vi "autofilter.vi"() -> ()   [LabVIEW 8.6]
uses:
  Controls/lxw_filter_criteria.ctl
  Controls/lxw_filter_operator.ctl
panel:
  out "error out":errorcluster
  out "function return 2":string
  # "autofilter.xlsx"
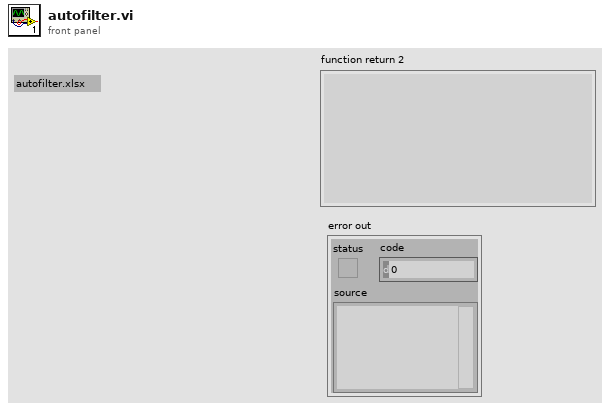
[diagram p1: front panel]
types:
  T1 = typedef "lxw_filter_operator.ctl" = u8
  T2 = typedef "lxw_filter_criteria.ctl" = u32
  T3 = cluster{"criteria":T2, "value_string":string, "value":dbl}
  T4 = cluster{"region":string[], "item":string[], "volume":i32[], "month":string[]}
  T5 = enum32{"invalid app kind", "Development System", "Run Time System", "Student Edition", "Embedded LabVIEW", "Evaluation", "Custom"}
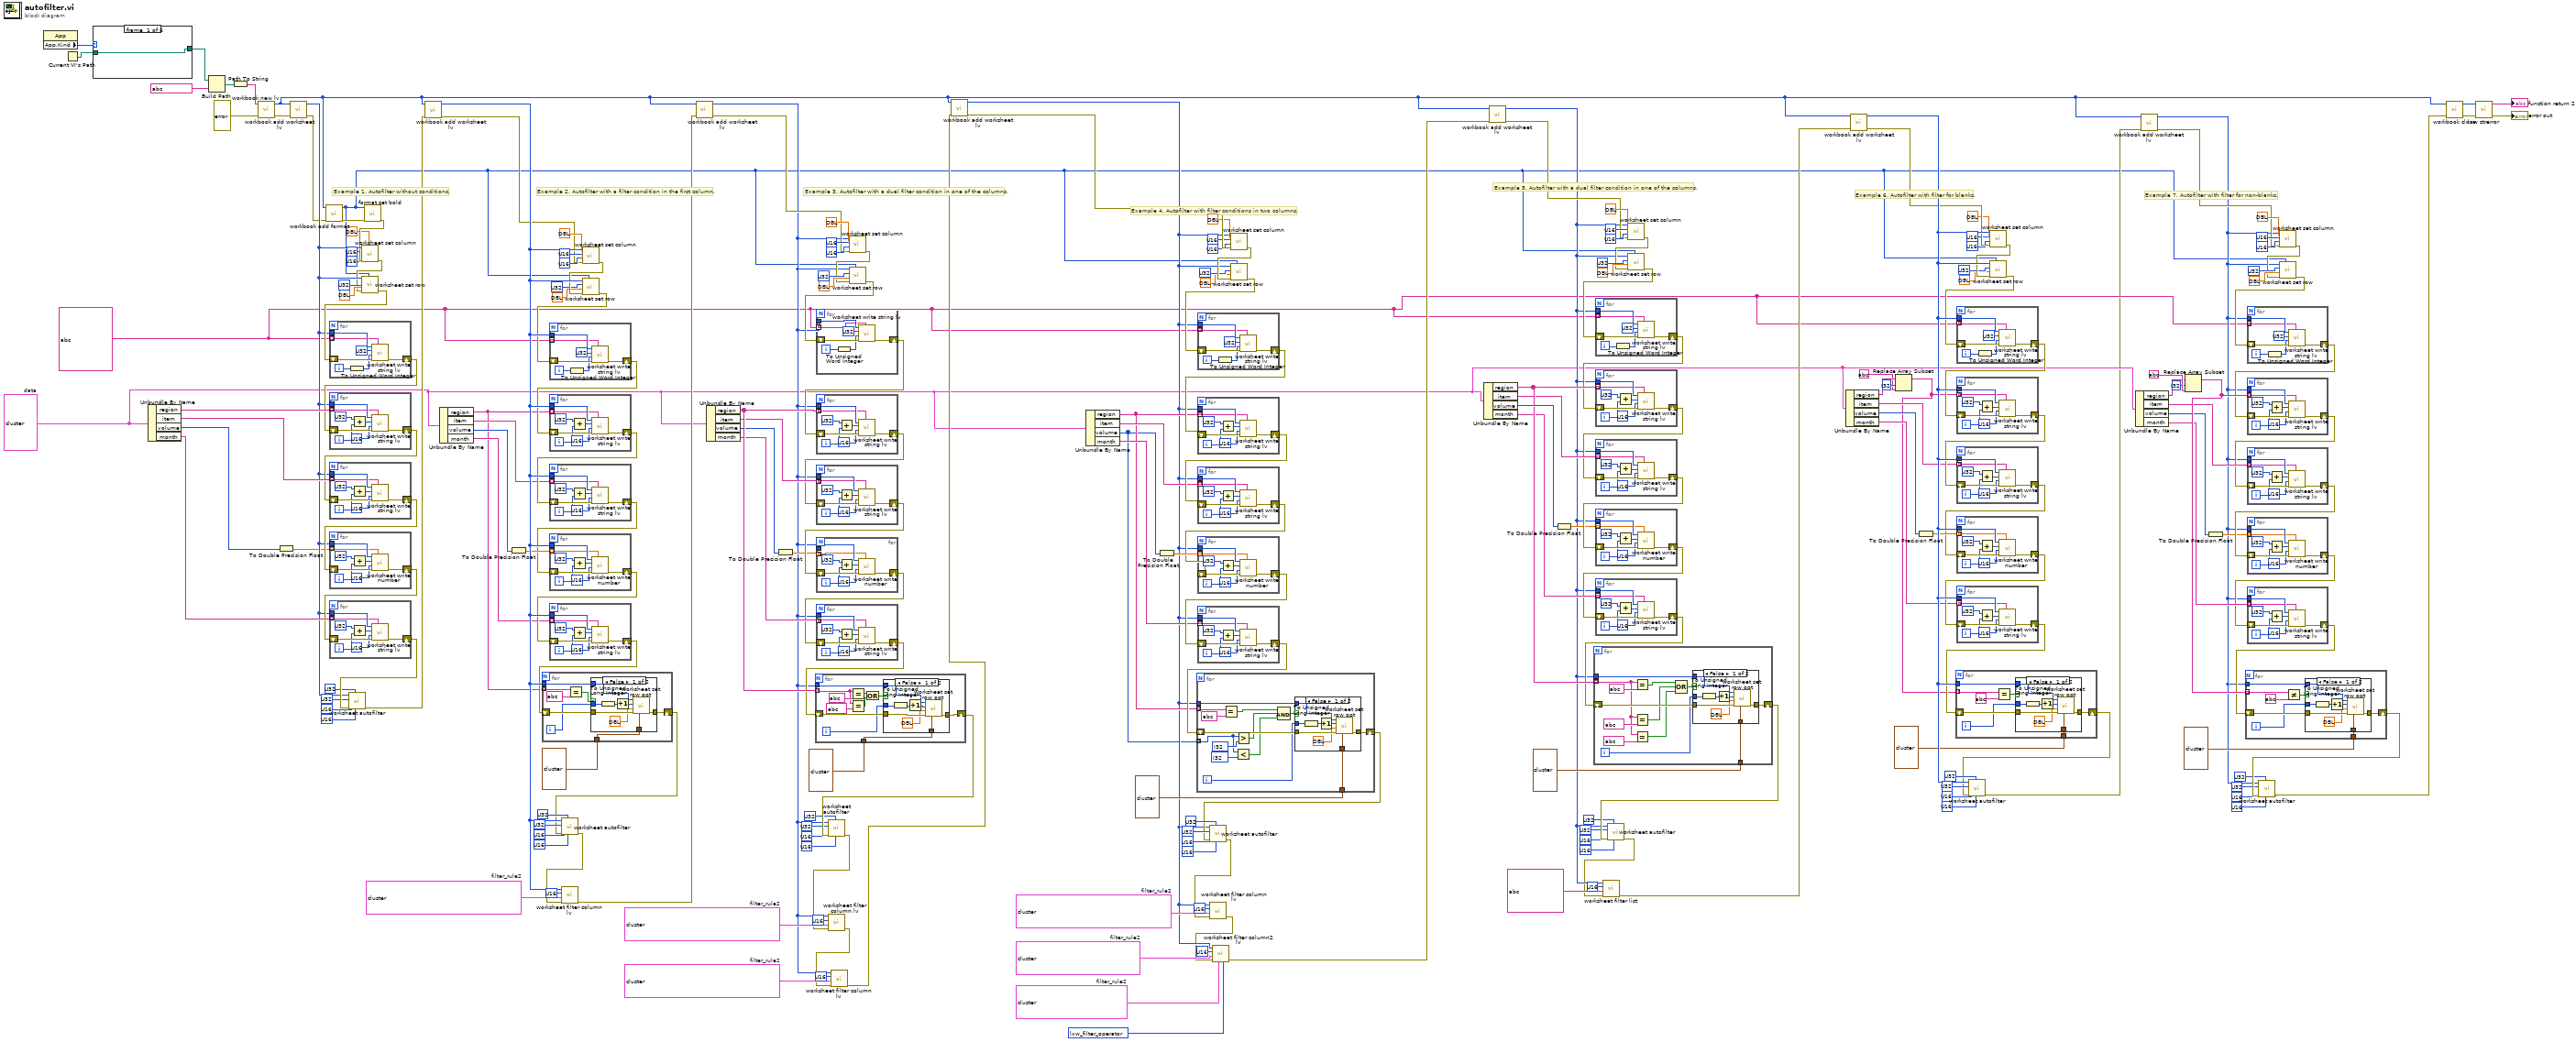
[diagram p0: block diagram]
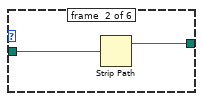
[diagram p8: hidden frame]
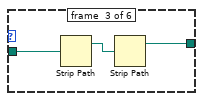
[diagram p9: hidden frame]
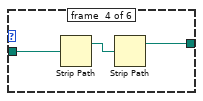
[diagram p10: hidden frame]
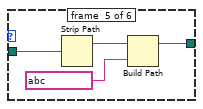
[diagram p11: hidden frame]
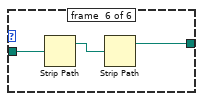
[diagram p12: hidden frame]
diagram:
  w95 = T1 ? items=["LXW_FILTER_AND", "LXW_FILTER_OR"] ("and_or")
  w97 = T3 ?  # filter_rule2
  w98 = T3 ?  # filter_rule2
  w103 = T3 ?  # filter_rule2
  w130 = T3 ?  # filter_rule2
  w155 = T3 ?  # filter_rule2
  w160 = T3 ?  # filter_rule2
  w5 = T4 ?  # data
  w6 = string[] ?
  # "Example 7. Autofilter with filter for non-blanks."
  # "Example 6. Autofilter with filter for blanks."
  # "Example 5. Autofilter with a dual filter condition in one of the columns."
  # "Example 4. Autofilter with filter conditions in two columns."
  # "Example 3. Autofilter with a dual filter condition in one of the columns."
  # "Example 2. Autofilter with a filter condition in the first column."
  # "Example 1. Autofilter without conditions."
  n1 = property class="App"() -> ("App.Kind"=w224:T5)  [unwired: 2 in, 2 out]
  n2 = Current VI's Path() -> (path=w223:path)
  n3 = case shown="\"Evaluation\"" w224 {
    tunnel: w223 -> [w225 w227 w230 w233 w237 w240]
    tunnel: [w225 w226 w228 w231 w235 w238] -> w222
    frame #0 {
    }
    frame #1 {
      n4 = Strip Path(path=w227) -> (stripped path=w226:path)  [unwired: 1 out]
    }
    frame #2 {
      n5 = Strip Path(path=w230) -> (stripped path=w229:path)  [unwired: 1 out]
      n6 = Strip Path(path=w229) -> (stripped path=w228:path)  [unwired: 1 out]
    }
    frame #3 {
      n7 = Strip Path(path=w233) -> (stripped path=w232:path)  [unwired: 1 out]
      n8 = Strip Path(path=w232) -> (stripped path=w231:path)  [unwired: 1 out]
    }
    frame #4 {
      n9 = Strip Path(path=w237) -> (stripped path=w236:path)  [unwired: 1 out]
      n10 = Build Path(base path=w236, name or relative path=string ?) -> (appended path=w235:path)
    }
    frame #5 {
      n11 = Strip Path(path=w240) -> (stripped path=w239:path)  [unwired: 1 out]
      n12 = Strip Path(path=w239) -> (stripped path=w238:path)  [unwired: 1 out]
    }
  }
  n13 = Unbundle By Name(w5) -> ("region"=w212:string[], "item"=w211:string[], "volume"=w202:i32[], "month"=w210:string[])
  n14 = Build Path(base path=w222, name or relative path=string ? ("filename")) -> (appended path=w214:path)
  n15 = Path To String(path=w214) -> (string=w213:string)
  n16 = call "workbook new lv.vi"("error in (no error)"=errorcluster ?, "filename"=w213) -> ("error out"=w220:errorcluster, "function return"=w4:u32)  [unwired: 8 in]
  n17 = To Double Precision Float(number=w202) -> (double precision float=w201:dbl[])
  n18 = call "workbook add worksheet lv.vi"("error in (no error)"=w220, "workbook"=w4) -> ("error out"=w199:errorcluster, "function return"=w203:u32)  [unwired: 8 in]
  n19 = call "workbook add format.vi"("error in (no error)"=w199, "workbook"=w4) -> ("error out"=w191:errorcluster, "function return"=w2:u32)  [unwired: 8 in]
  n20 = call "format set bold.vi"("error in (no error)"=w191, "format"=w2) -> ("error out"=w190:errorcluster)  [unwired: 9 in]
  n21 = call "worksheet set column.vi"("width"=dbl ?, "error in (no error)"=w190, "last_col"=u16 ?, "first_col"=u16 ?, "worksheet"=w203) -> ("error out"=w184:errorcluster)  [unwired: 5 in, 1 out]
  n22 = call "worksheet set row.vi"("format"=w2, "error in (no error)"=w184, "height"=dbl ?, "row"=u32 ?, "worksheet"=w203) -> ("error out"=w209:errorcluster)  [unwired: 5 in, 1 out]
  n23 = for {
    shift-right: [w247] -> w208
    shift-left: w209 -> [w246]
    tunnel: w203 -> [w245]
    tunnel: w6 -> [w244] mode=indexing
    i -> [w242]
    n24 = To Unsigned Word Integer(number=w242) -> (unsigned 16bit integer=w241:u16)
    n25 = call "worksheet write string lv.vi"("string"=w244, "error in (no error)"=w246, "col"=w241, "row"=u32 ?, "worksheet"=w245) -> ("error out"=w247:errorcluster)  [unwired: 5 in, 1 out]
  }
  n26 = for {
    shift-right: [w255] -> w207
    shift-left: w208 -> [w254]
    tunnel: w203 -> [w251]
    tunnel: w212 -> [w248] mode=indexing
    i -> [w250]
    n27 = Add(x=u32 ? ("row"), y=w250) -> (x+y=w253:u32)
    n28 = call "worksheet write string lv.vi"("string"=w248, "error in (no error)"=w254, "col"=u16 ?, "row"=w253, "worksheet"=w251) -> ("error out"=w255:errorcluster)  [unwired: 5 in, 1 out]
  }
  n29 = for {
    shift-right: [w263] -> w206
    shift-left: w207 -> [w262]
    tunnel: w203 -> [w259]
    tunnel: w211 -> [w256] mode=indexing
    i -> [w258]
    n30 = Add(x=u32 ? ("row"), y=w258) -> (x+y=w261:u32)
    n31 = call "worksheet write string lv.vi"("string"=w256, "error in (no error)"=w262, "col"=u16 ?, "row"=w261, "worksheet"=w259) -> ("error out"=w263:errorcluster)  [unwired: 5 in, 1 out]
  }
  n32 = for {
    shift-right: [w271] -> w205
    shift-left: w206 -> [w270]
    tunnel: w203 -> [w267]
    tunnel: w201 -> [w264] mode=indexing
    i -> [w266]
    n33 = Add(x=u32 ? ("row"), y=w266) -> (x+y=w269:u32)
    n34 = call "worksheet write number.vi"("number"=w264, "error in (no error)"=w270, "col"=u16 ?, "row"=w269, "worksheet"=w267) -> ("error out"=w271:errorcluster)  [unwired: 5 in, 1 out]
  }
  n35 = for {
    shift-right: [w279] -> w204
    shift-left: w205 -> [w278]
    tunnel: w203 -> [w275]
    tunnel: w210 -> [w272] mode=indexing
    i -> [w274]
    n36 = Add(x=u32 ? ("row"), y=w274) -> (x+y=w277:u32)
    n37 = call "worksheet write string lv.vi"("string"=w272, "error in (no error)"=w278, "col"=u16 ?, "row"=w277, "worksheet"=w275) -> ("error out"=w279:errorcluster)  [unwired: 5 in, 1 out]
  }
  n38 = call "worksheet autofilter.vi"("last_col"=u16 ?, "last_row"=u32 ?, "error in (no error)"=w204, "first_col"=u16 ?, "first_row"=u32 ?, "worksheet"=w203) -> ("error out"=w200:errorcluster)  [unwired: 4 in, 1 out]
  n39 = call "workbook add worksheet lv.vi"("error in (no error)"=w200, "workbook"=w4) -> ("error out"=w161:errorcluster, "function return"=w197:u32)  [unwired: 8 in]
  n40 = Unbundle By Name(w5) -> ("region"=w162:string[], "item"=w165:string[], "volume"=w182:i32[], "month"=w166:string[])
  n41 = To Double Precision Float(number=w182) -> (double precision float=w183:dbl[])
  n42 = call "worksheet set column.vi"("width"=dbl ?, "error in (no error)"=w161, "last_col"=u16 ?, "first_col"=u16 ?, "worksheet"=w197) -> ("error out"=w176:errorcluster)  [unwired: 5 in, 1 out]
  n43 = call "worksheet set row.vi"("format"=w2, "error in (no error)"=w176, "height"=dbl ?, "row"=u32 ?, "worksheet"=w197) -> ("error out"=w177:errorcluster)  [unwired: 5 in, 1 out]
  n44 = for {
    shift-right: [w286] -> w178
    shift-left: w177 -> [w285]
    tunnel: w197 -> [w284]
    tunnel: w6 -> [w283] mode=indexing
    i -> [w281]
    n45 = To Unsigned Word Integer(number=w281) -> (unsigned 16bit integer=w280:u16)
    n46 = call "worksheet write string lv.vi"("string"=w283, "error in (no error)"=w285, "col"=w280, "row"=u32 ?, "worksheet"=w284) -> ("error out"=w286:errorcluster)  [unwired: 5 in, 1 out]
  }
  n47 = for {
    shift-right: [w294] -> w179
    shift-left: w178 -> [w293]
    tunnel: w197 -> [w290]
    tunnel: w162 -> [w287] mode=indexing
    i -> [w289]
    n48 = Add(x=u32 ? ("row"), y=w289) -> (x+y=w292:u32)
    n49 = call "worksheet write string lv.vi"("string"=w287, "error in (no error)"=w293, "col"=u16 ?, "row"=w292, "worksheet"=w290) -> ("error out"=w294:errorcluster)  [unwired: 5 in, 1 out]
  }
  n50 = for {
    shift-right: [w302] -> w180
    shift-left: w179 -> [w301]
    tunnel: w197 -> [w298]
    tunnel: w165 -> [w295] mode=indexing
    i -> [w297]
    n51 = Add(x=u32 ? ("row"), y=w297) -> (x+y=w300:u32)
    n52 = call "worksheet write string lv.vi"("string"=w295, "error in (no error)"=w301, "col"=u16 ?, "row"=w300, "worksheet"=w298) -> ("error out"=w302:errorcluster)  [unwired: 5 in, 1 out]
  }
  n53 = for {
    shift-right: [w310] -> w181
    shift-left: w180 -> [w309]
    tunnel: w197 -> [w306]
    tunnel: w183 -> [w303] mode=indexing
    i -> [w305]
    n54 = Add(x=u32 ? ("row"), y=w305) -> (x+y=w308:u32)
    n55 = call "worksheet write number.vi"("number"=w303, "error in (no error)"=w309, "col"=u16 ?, "row"=w308, "worksheet"=w306) -> ("error out"=w310:errorcluster)  [unwired: 5 in, 1 out]
  }
  n56 = for {
    shift-right: [w318] -> w164
    shift-left: w181 -> [w317]
    tunnel: w197 -> [w314]
    tunnel: w166 -> [w311] mode=indexing
    i -> [w313]
    n57 = Add(x=u32 ? ("row"), y=w313) -> (x+y=w316:u32)
    n58 = call "worksheet write string lv.vi"("string"=w311, "error in (no error)"=w317, "col"=u16 ?, "row"=w316, "worksheet"=w314) -> ("error out"=w318:errorcluster)  [unwired: 5 in, 1 out]
  }
  n59 = for {
    shift-right: [w325] -> w163
    shift-left: w164 -> [w326]
    tunnel: cluster{"hidden":u8, "level":u8, "collapsed":u8} ? ("options") -> [w324]
    tunnel: w162 -> [w323] mode=indexing
    tunnel: w197 -> [w321]
    i -> [w320]
    n60 = Equal?(x=w323, y=string ?) -> (x = y?=w319:bool)
    n61 = case shown="False" w319 {
      tunnel: w326 -> [w334 w335]
      tunnel: [w333 w335] -> w325
      tunnel: w324 -> [w332 _]
      tunnel: w321 -> [w327 _]
      tunnel: w320 -> [w330 _]
      frame #0 {
        n62 = To Unsigned Long Integer(number=w330) -> (unsigned 32bit integer=w329:u32)
        n63 = Increment(x=w329) -> (x+1=w331:u32)
        n64 = call "worksheet set row opt.vi"("options"=w332, "error in (no error)"=w334, "height"=dbl ? ("LXW_DEF_ROW_HEIGHT"), "row"=w331, "worksheet"=w327) -> ("error out"=w333:errorcluster)  [unwired: 4 in, 2 out]
      }
      frame #1 {
      }
    }
  }
  n65 = call "worksheet autofilter.vi"("last_col"=u16 ?, "last_row"=u32 ?, "error in (no error)"=w163, "first_col"=u16 ?, "first_row"=u32 ?, "worksheet"=w197) -> ("error out"=w196:errorcluster)  [unwired: 4 in, 1 out]
  n66 = call "worksheet filter column lv.vi"("error in (no error)"=w196, "lxw_filter_rule"=w160, "col"=u16 ?, "worksheet"=w197) -> ("error out"=w198:errorcluster)  [unwired: 5 in, 2 out]
  n67 = call "workbook add worksheet lv.vi"("error in (no error)"=w198, "workbook"=w4) -> ("error out"=w131:errorcluster, "function return"=w127:u32)  [unwired: 8 in]
  n68 = Unbundle By Name(w5) -> ("region"=w154:string[], "item"=w151:string[], "volume"=w134:i32[], "month"=w150:string[])
  n69 = To Double Precision Float(number=w134) -> (double precision float=w133:dbl[])
  n70 = call "worksheet set column.vi"("width"=dbl ?, "error in (no error)"=w131, "last_col"=u16 ?, "first_col"=u16 ?, "worksheet"=w127) -> ("error out"=w140:errorcluster)  [unwired: 5 in, 1 out]
  n71 = call "worksheet set row.vi"("format"=w2, "error in (no error)"=w140, "height"=dbl ?, "row"=u32 ?, "worksheet"=w127) -> ("error out"=w139:errorcluster)  [unwired: 5 in, 1 out]
  n72 = for {
    shift-right: [w342] -> w138
    shift-left: w139 -> [w341]
    tunnel: w127 -> [w340]
    tunnel: w6 -> [w339] mode=indexing
    i -> [w337]
    n73 = To Unsigned Word Integer(number=w337) -> (unsigned 16bit integer=w336:u16)
    n74 = call "worksheet write string lv.vi"("string"=w339, "error in (no error)"=w341, "col"=w336, "row"=u32 ?, "worksheet"=w340) -> ("error out"=w342:errorcluster)  [unwired: 5 in, 1 out]
  }
  n75 = for {
    shift-right: [w350] -> w137
    shift-left: w138 -> [w349]
    tunnel: w127 -> [w346]
    tunnel: w154 -> [w343] mode=indexing
    i -> [w345]
    n76 = Add(x=u32 ? ("row"), y=w345) -> (x+y=w348:u32)
    n77 = call "worksheet write string lv.vi"("string"=w343, "error in (no error)"=w349, "col"=u16 ?, "row"=w348, "worksheet"=w346) -> ("error out"=w350:errorcluster)  [unwired: 5 in, 1 out]
  }
  n78 = for {
    shift-right: [w358] -> w136
    shift-left: w137 -> [w357]
    tunnel: w127 -> [w354]
    tunnel: w151 -> [w351] mode=indexing
    i -> [w353]
    n79 = Add(x=u32 ? ("row"), y=w353) -> (x+y=w356:u32)
    n80 = call "worksheet write string lv.vi"("string"=w351, "error in (no error)"=w357, "col"=u16 ?, "row"=w356, "worksheet"=w354) -> ("error out"=w358:errorcluster)  [unwired: 5 in, 1 out]
  }
  n81 = for {
    shift-right: [w366] -> w135
    shift-left: w136 -> [w365]
    tunnel: w127 -> [w362]
    tunnel: w133 -> [w359] mode=indexing
    i -> [w361]
    n82 = Add(x=u32 ? ("row"), y=w361) -> (x+y=w364:u32)
    n83 = call "worksheet write number.vi"("number"=w359, "error in (no error)"=w365, "col"=u16 ?, "row"=w364, "worksheet"=w362) -> ("error out"=w366:errorcluster)  [unwired: 5 in, 1 out]
  }
  n84 = for {
    shift-right: [w374] -> w152
    shift-left: w135 -> [w373]
    tunnel: w127 -> [w370]
    tunnel: w150 -> [w367] mode=indexing
    i -> [w369]
    n85 = Add(x=u32 ? ("row"), y=w369) -> (x+y=w372:u32)
    n86 = call "worksheet write string lv.vi"("string"=w367, "error in (no error)"=w373, "col"=u16 ?, "row"=w372, "worksheet"=w370) -> ("error out"=w374:errorcluster)  [unwired: 5 in, 1 out]
  }
  n87 = for {
    shift-right: [w384] -> w153
    shift-left: w152 -> [w385]
    tunnel: cluster{"hidden":u8, "level":u8, "collapsed":u8} ? ("options") -> [w383]
    tunnel: w154 -> [w379] mode=indexing
    tunnel: w127 -> [w382]
    i -> [w381]
    n88 = Equal?(x=w379, y=string ?) -> (x = y?=w376:bool)
    n89 = Equal?(x=w379, y=string ?) -> (x = y?=w375:bool)
    n90 = Or(x=w376, y=w375) -> (x .or. y?=w377:bool)
    n91 = case shown="False" w377 {
      tunnel: w385 -> [w393 w394]
      tunnel: [w392 w394] -> w384
      tunnel: w383 -> [w391 _]
      tunnel: w382 -> [w386 _]
      tunnel: w381 -> [w389 _]
      frame #0 {
        n92 = To Unsigned Long Integer(number=w389) -> (unsigned 32bit integer=w388:u32)
        n93 = Increment(x=w388) -> (x+1=w390:u32)
        n94 = call "worksheet set row opt.vi"("options"=w391, "error in (no error)"=w393, "height"=dbl ? ("LXW_DEF_ROW_HEIGHT"), "row"=w390, "worksheet"=w386) -> ("error out"=w392:errorcluster)  [unwired: 4 in, 2 out]
      }
      frame #1 {
      }
    }
  }
  n95 = call "worksheet autofilter.vi"("last_col"=u16 ?, "last_row"=u32 ?, "error in (no error)"=w153, "first_col"=u16 ?, "first_row"=u32 ?, "worksheet"=w127) -> ("error out"=w132:errorcluster)  [unwired: 4 in, 1 out]
  n96 = call "worksheet filter column lv.vi"("error in (no error)"=w132, "lxw_filter_rule"=w155, "col"=u16 ?, "worksheet"=w127) -> ("error out"=w128:errorcluster)  [unwired: 5 in, 2 out]
  n97 = call "worksheet filter column lv.vi"("error in (no error)"=w128, "lxw_filter_rule"=w130, "col"=u16 ?, "worksheet"=w127) -> ("error out"=w100:errorcluster)  [unwired: 5 in, 2 out]
  n98 = call "workbook add worksheet lv.vi"("error in (no error)"=w100, "workbook"=w4) -> ("error out"=w126:errorcluster, "function return"=w99:u32)  [unwired: 8 in]
  n99 = Unbundle By Name(w5) -> ("region"=w104:string[], "item"=w107:string[], "volume"=w93:i32[], "month"=w108:string[])
  n100 = To Double Precision Float(number=w93) -> (double precision float=w124:dbl[])
  n101 = call "worksheet set column.vi"("width"=dbl ?, "error in (no error)"=w126, "last_col"=u16 ?, "first_col"=u16 ?, "worksheet"=w99) -> ("error out"=w118:errorcluster)  [unwired: 5 in, 1 out]
  n102 = call "worksheet set row.vi"("format"=w2, "error in (no error)"=w118, "height"=dbl ?, "row"=u32 ?, "worksheet"=w99) -> ("error out"=w119:errorcluster)  [unwired: 5 in, 1 out]
  n103 = for {
    shift-right: [w401] -> w120
    shift-left: w119 -> [w400]
    tunnel: w99 -> [w399]
    tunnel: w6 -> [w398] mode=indexing
    i -> [w396]
    n104 = To Unsigned Word Integer(number=w396) -> (unsigned 16bit integer=w395:u16)
    n105 = call "worksheet write string lv.vi"("string"=w398, "error in (no error)"=w400, "col"=w395, "row"=u32 ?, "worksheet"=w399) -> ("error out"=w401:errorcluster)  [unwired: 5 in, 1 out]
  }
  n106 = for {
    shift-right: [w409] -> w121
    shift-left: w120 -> [w408]
    tunnel: w99 -> [w405]
    tunnel: w104 -> [w402] mode=indexing
    i -> [w404]
    n107 = Add(x=u32 ? ("row"), y=w404) -> (x+y=w407:u32)
    n108 = call "worksheet write string lv.vi"("string"=w402, "error in (no error)"=w408, "col"=u16 ?, "row"=w407, "worksheet"=w405) -> ("error out"=w409:errorcluster)  [unwired: 5 in, 1 out]
  }
  n109 = for {
    shift-right: [w417] -> w122
    shift-left: w121 -> [w416]
    tunnel: w99 -> [w413]
    tunnel: w107 -> [w410] mode=indexing
    i -> [w412]
    n110 = Add(x=u32 ? ("row"), y=w412) -> (x+y=w415:u32)
    n111 = call "worksheet write string lv.vi"("string"=w410, "error in (no error)"=w416, "col"=u16 ?, "row"=w415, "worksheet"=w413) -> ("error out"=w417:errorcluster)  [unwired: 5 in, 1 out]
  }
  n112 = for {
    shift-right: [w425] -> w123
    shift-left: w122 -> [w424]
    tunnel: w99 -> [w421]
    tunnel: w124 -> [w418] mode=indexing
    i -> [w420]
    n113 = Add(x=u32 ? ("row"), y=w420) -> (x+y=w423:u32)
    n114 = call "worksheet write number.vi"("number"=w418, "error in (no error)"=w424, "col"=u16 ?, "row"=w423, "worksheet"=w421) -> ("error out"=w425:errorcluster)  [unwired: 5 in, 1 out]
  }
  n115 = for {
    shift-right: [w433] -> w106
    shift-left: w123 -> [w432]
    tunnel: w99 -> [w429]
    tunnel: w108 -> [w426] mode=indexing
    i -> [w428]
    n116 = Add(x=u32 ? ("row"), y=w428) -> (x+y=w431:u32)
    n117 = call "worksheet write string lv.vi"("string"=w426, "error in (no error)"=w432, "col"=u16 ?, "row"=w431, "worksheet"=w429) -> ("error out"=w433:errorcluster)  [unwired: 5 in, 1 out]
  }
  n118 = for {
    shift-right: [w446] -> w105
    shift-left: w106 -> [w447]
    tunnel: cluster{"hidden":u8, "level":u8, "collapsed":u8} ? ("options") -> [w440]
    tunnel: w104 -> [w443] mode=indexing
    tunnel: w99 -> [w445]
    tunnel: w93 -> [w435] mode=indexing
    i -> [w439]
    n119 = Equal?(x=w443, y=string ?) -> (x = y?=w441:bool)
    n120 = Less?(x=w435, y=i32 ?) -> (x < y?=w437:bool)
    n121 = Greater?(x=w435, y=i32 ?) -> (0:w438:bool)
    n122 = Compound Arithmetic op=AND(w441, w438, w437) -> (w442:bool)
    n123 = case shown="False" w442 {
      tunnel: w447 -> [w455 w456]
      tunnel: [w454 w456] -> w446
      tunnel: w440 -> [w453 _]
      tunnel: w445 -> [w448 _]
      tunnel: w439 -> [w451 _]
      frame #0 {
        n124 = To Unsigned Long Integer(number=w451) -> (unsigned 32bit integer=w450:u32)
        n125 = Increment(x=w450) -> (x+1=w452:u32)
        n126 = call "worksheet set row opt.vi"("options"=w453, "error in (no error)"=w455, "height"=dbl ? ("LXW_DEF_ROW_HEIGHT"), "row"=w452, "worksheet"=w448) -> ("error out"=w454:errorcluster)  [unwired: 4 in, 2 out]
      }
      frame #1 {
      }
    }
  }
  n127 = call "worksheet autofilter.vi"("last_col"=u16 ?, "last_row"=u32 ?, "error in (no error)"=w105, "first_col"=u16 ?, "first_row"=u32 ?, "worksheet"=w99) -> ("error out"=w125:errorcluster)  [unwired: 4 in, 1 out]
  n128 = call "worksheet filter column lv.vi"("error in (no error)"=w125, "lxw_filter_rule"=w103, "col"=u16 ?, "worksheet"=w99) -> ("error out"=w96:errorcluster)  [unwired: 5 in, 2 out]
  n129 = call "worksheet filter column2 lv.vi"("and_or"=w95, "lxw_filter_rule 2"=w97, "error in (no error)"=w96, "lxw_filter_rule"=w98, "col"=u16 ?, "worksheet"=w99) -> ("error out"=w65:errorcluster)  [unwired: 4 in, 1 out]
  n130 = Unbundle By Name(w5) -> ("region"=w90:string[], "item"=w87:string[], "volume"=w92:i32[], "month"=w86:string[])
  n131 = call "workbook add worksheet lv.vi"("error in (no error)"=w65, "workbook"=w4) -> ("error out"=w69:errorcluster, "function return"=w67:u32)  [unwired: 8 in]
  n132 = To Double Precision Float(number=w92) -> (double precision float=w70:dbl[])
  n133 = call "worksheet set column.vi"("width"=dbl ?, "error in (no error)"=w69, "last_col"=u16 ?, "first_col"=u16 ?, "worksheet"=w67) -> ("error out"=w76:errorcluster)  [unwired: 5 in, 1 out]
  n134 = call "worksheet set row.vi"("format"=w2, "error in (no error)"=w76, "height"=dbl ?, "row"=u32 ?, "worksheet"=w67) -> ("error out"=w75:errorcluster)  [unwired: 5 in, 1 out]
  n135 = for {
    shift-right: [w463] -> w74
    shift-left: w75 -> [w462]
    tunnel: w67 -> [w461]
    tunnel: w6 -> [w460] mode=indexing
    i -> [w458]
    n136 = To Unsigned Word Integer(number=w458) -> (unsigned 16bit integer=w457:u16)
    n137 = call "worksheet write string lv.vi"("string"=w460, "error in (no error)"=w462, "col"=w457, "row"=u32 ?, "worksheet"=w461) -> ("error out"=w463:errorcluster)  [unwired: 5 in, 1 out]
  }
  n138 = for {
    shift-right: [w471] -> w73
    shift-left: w74 -> [w470]
    tunnel: w67 -> [w467]
    tunnel: w90 -> [w464] mode=indexing
    i -> [w466]
    n139 = Add(x=u32 ? ("row"), y=w466) -> (x+y=w469:u32)
    n140 = call "worksheet write string lv.vi"("string"=w464, "error in (no error)"=w470, "col"=u16 ?, "row"=w469, "worksheet"=w467) -> ("error out"=w471:errorcluster)  [unwired: 5 in, 1 out]
  }
  n141 = for {
    shift-right: [w479] -> w72
    shift-left: w73 -> [w478]
    tunnel: w67 -> [w475]
    tunnel: w87 -> [w472] mode=indexing
    i -> [w474]
    n142 = Add(x=u32 ? ("row"), y=w474) -> (x+y=w477:u32)
    n143 = call "worksheet write string lv.vi"("string"=w472, "error in (no error)"=w478, "col"=u16 ?, "row"=w477, "worksheet"=w475) -> ("error out"=w479:errorcluster)  [unwired: 5 in, 1 out]
  }
  n144 = for {
    shift-right: [w487] -> w71
    shift-left: w72 -> [w486]
    tunnel: w67 -> [w483]
    tunnel: w70 -> [w480] mode=indexing
    i -> [w482]
    n145 = Add(x=u32 ? ("row"), y=w482) -> (x+y=w485:u32)
    n146 = call "worksheet write number.vi"("number"=w480, "error in (no error)"=w486, "col"=u16 ?, "row"=w485, "worksheet"=w483) -> ("error out"=w487:errorcluster)  [unwired: 5 in, 1 out]
  }
  n147 = for {
    shift-right: [w495] -> w88
    shift-left: w71 -> [w494]
    tunnel: w67 -> [w491]
    tunnel: w86 -> [w488] mode=indexing
    i -> [w490]
    n148 = Add(x=u32 ? ("row"), y=w490) -> (x+y=w493:u32)
    n149 = call "worksheet write string lv.vi"("string"=w488, "error in (no error)"=w494, "col"=u16 ?, "row"=w493, "worksheet"=w491) -> ("error out"=w495:errorcluster)  [unwired: 5 in, 1 out]
  }
  n150 = for {
    shift-right: [w507] -> w89
    shift-left: w88 -> [w508]
    tunnel: cluster{"hidden":u8, "level":u8, "collapsed":u8} ? ("options") -> [w502]
    tunnel: w90 -> [w496] mode=indexing
    tunnel: w67 -> [w506]
    i -> [w501]
    n151 = Equal?(x=w496, y=string ?) -> (x = y?=w503:bool)
    n152 = Equal?(x=w496, y=string ?) -> (x = y?=w498:bool)
    n153 = Equal?(x=w496, y=string ?) -> (x = y?=w497:bool)
    n154 = Compound Arithmetic op=OR(w503, w498, w497) -> (w504:bool)
    n155 = case shown="False" w504 {
      tunnel: w508 -> [w516 w517]
      tunnel: [w515 w517] -> w507
      tunnel: w502 -> [w514 _]
      tunnel: w506 -> [w509 _]
      tunnel: w501 -> [w512 _]
      frame #0 {
        n156 = To Unsigned Long Integer(number=w512) -> (unsigned 32bit integer=w511:u32)
        n157 = Increment(x=w511) -> (x+1=w513:u32)
        n158 = call "worksheet set row opt.vi"("options"=w514, "error in (no error)"=w516, "height"=dbl ? ("LXW_DEF_ROW_HEIGHT"), "row"=w513, "worksheet"=w509) -> ("error out"=w515:errorcluster)  [unwired: 4 in, 2 out]
      }
      frame #1 {
      }
    }
  }
  n159 = call "worksheet autofilter.vi"("last_col"=u16 ?, "last_row"=u32 ?, "error in (no error)"=w89, "first_col"=u16 ?, "first_row"=u32 ?, "worksheet"=w67) -> ("error out"=w66:errorcluster)  [unwired: 4 in, 1 out]
  n160 = call "worksheet filter list.vi"("error in (no error)"=w66, "list"=string[] ?, "col"=u16 ?, "worksheet"=w67) -> ("error out"=w38:errorcluster)  [unwired: 6 in, 1 out]
  n161 = Unbundle By Name(w5) -> ("region"=w41:string[], "item"=w44:string[], "volume"=w39:i32[], "month"=w45:string[])
  n162 = call "workbook add worksheet lv.vi"("error in (no error)"=w38, "workbook"=w4) -> ("error out"=w62:errorcluster, "function return"=w63:u32)  [unwired: 8 in]
  n163 = Replace Array Subset(array=w41, new element=string ?, index=i32 ?) -> (w35:string[])
  n164 = To Double Precision Float(number=w39) -> (double precision float=w61:dbl[])
  n165 = call "worksheet set column.vi"("width"=dbl ?, "error in (no error)"=w62, "last_col"=u16 ?, "first_col"=u16 ?, "worksheet"=w63) -> ("error out"=w55:errorcluster)  [unwired: 5 in, 1 out]
  n166 = call "worksheet set row.vi"("format"=w2, "error in (no error)"=w55, "height"=dbl ?, "row"=u32 ?, "worksheet"=w63) -> ("error out"=w56:errorcluster)  [unwired: 5 in, 1 out]
  n167 = for {
    shift-right: [w524] -> w57
    shift-left: w56 -> [w523]
    tunnel: w63 -> [w522]
    tunnel: w6 -> [w521] mode=indexing
    i -> [w519]
    n168 = To Unsigned Word Integer(number=w519) -> (unsigned 16bit integer=w518:u16)
    n169 = call "worksheet write string lv.vi"("string"=w521, "error in (no error)"=w523, "col"=w518, "row"=u32 ?, "worksheet"=w522) -> ("error out"=w524:errorcluster)  [unwired: 5 in, 1 out]
  }
  n170 = for {
    shift-right: [w532] -> w58
    shift-left: w57 -> [w531]
    tunnel: w63 -> [w528]
    tunnel: w35 -> [w525] mode=indexing
    i -> [w527]
    n171 = Add(x=u32 ? ("row"), y=w527) -> (x+y=w530:u32)
    n172 = call "worksheet write string lv.vi"("string"=w525, "error in (no error)"=w531, "col"=u16 ?, "row"=w530, "worksheet"=w528) -> ("error out"=w532:errorcluster)  [unwired: 5 in, 1 out]
  }
  n173 = for {
    shift-right: [w540] -> w59
    shift-left: w58 -> [w539]
    tunnel: w63 -> [w536]
    tunnel: w44 -> [w533] mode=indexing
    i -> [w535]
    n174 = Add(x=u32 ? ("row"), y=w535) -> (x+y=w538:u32)
    n175 = call "worksheet write string lv.vi"("string"=w533, "error in (no error)"=w539, "col"=u16 ?, "row"=w538, "worksheet"=w536) -> ("error out"=w540:errorcluster)  [unwired: 5 in, 1 out]
  }
  n176 = for {
    shift-right: [w548] -> w60
    shift-left: w59 -> [w547]
    tunnel: w63 -> [w544]
    tunnel: w61 -> [w541] mode=indexing
    i -> [w543]
    n177 = Add(x=u32 ? ("row"), y=w543) -> (x+y=w546:u32)
    n178 = call "worksheet write number.vi"("number"=w541, "error in (no error)"=w547, "col"=u16 ?, "row"=w546, "worksheet"=w544) -> ("error out"=w548:errorcluster)  [unwired: 5 in, 1 out]
  }
  n179 = for {
    shift-right: [w556] -> w43
    shift-left: w60 -> [w555]
    tunnel: w63 -> [w552]
    tunnel: w45 -> [w549] mode=indexing
    i -> [w551]
    n180 = Add(x=u32 ? ("row"), y=w551) -> (x+y=w554:u32)
    n181 = call "worksheet write string lv.vi"("string"=w549, "error in (no error)"=w555, "col"=u16 ?, "row"=w554, "worksheet"=w552) -> ("error out"=w556:errorcluster)  [unwired: 5 in, 1 out]
  }
  n182 = for {
    shift-right: [w563] -> w42
    shift-left: w43 -> [w564]
    tunnel: cluster{"hidden":u8, "level":u8, "collapsed":u8} ? ("options") -> [w560]
    tunnel: w35 -> [w559] mode=indexing
    tunnel: w63 -> [w562]
    i -> [w557]
    n183 = Equal?(x=w559, y=string ?) -> (x = y?=w558:bool)
    n184 = case shown="False" w558 {
      tunnel: w564 -> [w572 w573]
      tunnel: [w571 w573] -> w563
      tunnel: w560 -> [w570 _]
      tunnel: w562 -> [w565 _]
      tunnel: w557 -> [w568 _]
      frame #0 {
        n185 = To Unsigned Long Integer(number=w568) -> (unsigned 32bit integer=w567:u32)
        n186 = Increment(x=w567) -> (x+1=w569:u32)
        n187 = call "worksheet set row opt.vi"("options"=w570, "error in (no error)"=w572, "height"=dbl ? ("LXW_DEF_ROW_HEIGHT"), "row"=w569, "worksheet"=w565) -> ("error out"=w571:errorcluster)  [unwired: 4 in, 2 out]
      }
      frame #1 {
      }
    }
  }
  n188 = call "worksheet autofilter.vi"("last_col"=u16 ?, "last_row"=u32 ?, "error in (no error)"=w42, "first_col"=u16 ?, "first_row"=u32 ?, "worksheet"=w63) -> ("error out"=w3:errorcluster)  [unwired: 4 in, 1 out]
  n189 = Unbundle By Name(w5) -> ("region"=w29:string[], "item"=w26:string[], "volume"=w31:i32[], "month"=w25:string[])
  n190 = call "workbook add worksheet lv.vi"("error in (no error)"=w3, "workbook"=w4) -> ("error out"=w8:errorcluster, "function return"=w7:u32)  [unwired: 8 in]
  n191 = Replace Array Subset(array=w29, new element=string ?, index=i32 ?) -> (w34:string[])
  n192 = To Double Precision Float(number=w31) -> (double precision float=w9:dbl[])
  n193 = call "worksheet set column.vi"("width"=dbl ?, "error in (no error)"=w8, "last_col"=u16 ?, "first_col"=u16 ?, "worksheet"=w7) -> ("error out"=w15:errorcluster)  [unwired: 5 in, 1 out]
  n194 = call "worksheet set row.vi"("format"=w2, "error in (no error)"=w15, "height"=dbl ?, "row"=u32 ?, "worksheet"=w7) -> ("error out"=w14:errorcluster)  [unwired: 5 in, 1 out]
  n195 = for {
    shift-right: [w580] -> w13
    shift-left: w14 -> [w579]
    tunnel: w7 -> [w578]
    tunnel: w6 -> [w577] mode=indexing
    i -> [w575]
    n196 = To Unsigned Word Integer(number=w575) -> (unsigned 16bit integer=w574:u16)
    n197 = call "worksheet write string lv.vi"("string"=w577, "error in (no error)"=w579, "col"=w574, "row"=u32 ?, "worksheet"=w578) -> ("error out"=w580:errorcluster)  [unwired: 5 in, 1 out]
  }
  n198 = for {
    shift-right: [w588] -> w12
    shift-left: w13 -> [w587]
    tunnel: w7 -> [w584]
    tunnel: w34 -> [w581] mode=indexing
    i -> [w583]
    n199 = Add(x=u32 ? ("row"), y=w583) -> (x+y=w586:u32)
    n200 = call "worksheet write string lv.vi"("string"=w581, "error in (no error)"=w587, "col"=u16 ?, "row"=w586, "worksheet"=w584) -> ("error out"=w588:errorcluster)  [unwired: 5 in, 1 out]
  }
  n201 = for {
    shift-right: [w596] -> w11
    shift-left: w12 -> [w595]
    tunnel: w7 -> [w592]
    tunnel: w26 -> [w589] mode=indexing
    i -> [w591]
    n202 = Add(x=u32 ? ("row"), y=w591) -> (x+y=w594:u32)
    n203 = call "worksheet write string lv.vi"("string"=w589, "error in (no error)"=w595, "col"=u16 ?, "row"=w594, "worksheet"=w592) -> ("error out"=w596:errorcluster)  [unwired: 5 in, 1 out]
  }
  n204 = for {
    shift-right: [w604] -> w10
    shift-left: w11 -> [w603]
    tunnel: w7 -> [w600]
    tunnel: w9 -> [w597] mode=indexing
    i -> [w599]
    n205 = Add(x=u32 ? ("row"), y=w599) -> (x+y=w602:u32)
    n206 = call "worksheet write number.vi"("number"=w597, "error in (no error)"=w603, "col"=u16 ?, "row"=w602, "worksheet"=w600) -> ("error out"=w604:errorcluster)  [unwired: 5 in, 1 out]
  }
  n207 = for {
    shift-right: [w612] -> w27
    shift-left: w10 -> [w611]
    tunnel: w7 -> [w608]
    tunnel: w25 -> [w605] mode=indexing
    i -> [w607]
    n208 = Add(x=u32 ? ("row"), y=w607) -> (x+y=w610:u32)
    n209 = call "worksheet write string lv.vi"("string"=w605, "error in (no error)"=w611, "col"=u16 ?, "row"=w610, "worksheet"=w608) -> ("error out"=w612:errorcluster)  [unwired: 5 in, 1 out]
  }
  n210 = for {
    shift-right: [w619] -> w28
    shift-left: w27 -> [w620]
    tunnel: cluster{"hidden":u8, "level":u8, "collapsed":u8} ? ("options") -> [w616]
    tunnel: w34 -> [w615] mode=indexing
    tunnel: w7 -> [w618]
    i -> [w613]
    n211 = Not Equal?(x=w615, y=string ?) -> (x != y?=w614:bool)
    n212 = case shown="False" w614 {
      tunnel: w620 -> [w628 w629]
      tunnel: [w627 w629] -> w619
      tunnel: w616 -> [w626 _]
      tunnel: w618 -> [w621 _]
      tunnel: w613 -> [w624 _]
      frame #0 {
        n213 = To Unsigned Long Integer(number=w624) -> (unsigned 32bit integer=w623:u32)
        n214 = Increment(x=w623) -> (x+1=w625:u32)
        n215 = call "worksheet set row opt.vi"("options"=w626, "error in (no error)"=w628, "height"=dbl ? ("LXW_DEF_ROW_HEIGHT"), "row"=w625, "worksheet"=w621) -> ("error out"=w627:errorcluster)  [unwired: 4 in, 2 out]
      }
      frame #1 {
      }
    }
  }
  n216 = call "worksheet autofilter.vi"("last_col"=u16 ?, "last_row"=u32 ?, "error in (no error)"=w28, "first_col"=u16 ?, "first_row"=u32 ?, "worksheet"=w7) -> ("error out"=w1:errorcluster)  [unwired: 4 in, 1 out]
  n217 = call "workbook close.vi"("error in (no error)"=w1, "workbook"=w4) -> ("error out"=w216:errorcluster, "function return"=w218:u32)  [unwired: 8 in]
  n218 = call "lxw strerror.vi"("error in (no error)"=w216, "error_num"=w218) -> ("error out"=→"error out":errorcluster, "function return"=→"function return 2":string)  [unwired: 8 in]
